vi "RecorderMain.vi"(2 "Timer (Timer 1)":T1 items=["Timer 1", "Timer 2", "Timer 3"], 5 "NXT":T2={"Hardware"="NXT", "Flattened String"=""}) -> ()   [LabVIEW 2010, in "Recorder.lvlib"]
uses:
  Recorder.lvlib
  <vilib>/NXT/Subs/LVHSConnector.ctl
  <vilib>/NXT/Block Support/NXT_TimerIndex.ctl
  <vilib>/NXT/Dual Mode Library/Waits/Wait_Num(msec).vi
  Components/Components.lvlib
panel:
  out "LastWriterPowers":i16[](array[numeric])
  out "TeleopEnabled":bool
  out "Stop Program?":bool
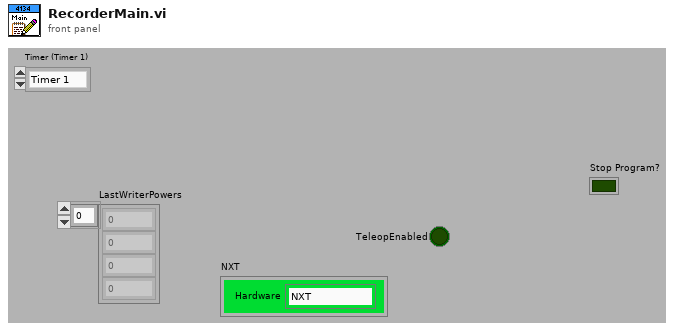
[diagram p1: front panel]
types:
  T1 = typedef "NXT_TimerIndex.ctl" = u8
  T2 = typedef "LVHSConnector.ctl" = cluster{"Hardware":string, "Flattened String":string}
  T3 = cluster{"FileName":string, "WriterEnabled?":bool, "TeleopEnabled?":bool, "StopProgram?":bool, "ArraySize":u8}
  T4 = typedef "NXT_FileStatusCodes.ctl" = u16
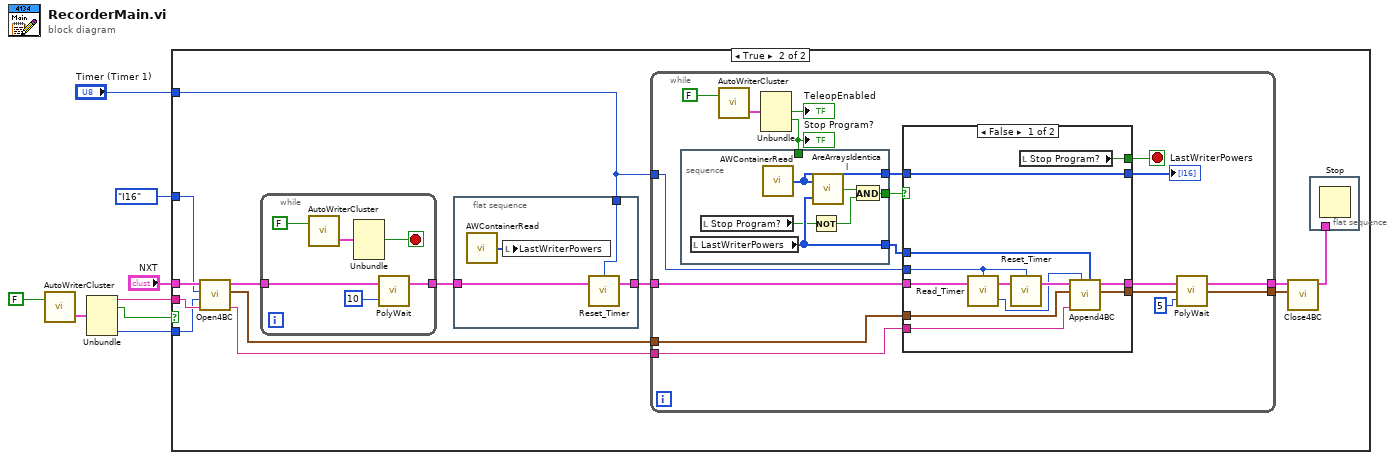
[diagram p0: block diagram]
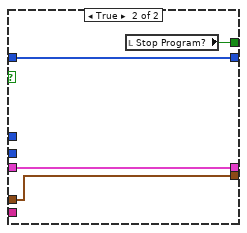
[diagram p3: hidden frame]
diagram:
  n1 = call "AutoWriterCluster.vi"("Mode(Write=True)"=FALSE) -> ("Output"=w7:T3)  [unwired: 1 in]
  n2 = Unbundle(w7) -> ("FileName"=w5:string, "WriterEnabled?"=w6:bool, "ArraySize"=w4:u8)  [unwired: 2 out]
  n3 = case shown="True" w6 {
    tunnel: w5 -> [_ w18]
    tunnel: w4 -> [_ w17]
    tunnel: "NXT" -> [_ w16]
    tunnel: "Timer (Timer 1)" -> [_ w15]
    tunnel: enum8{"I8", "I16"}."I16" ("Storage Size (I16)") -> [_ w10]
    frame False {
    }
    frame True {
      n4 = call "Open4BC.vi"("File"=w18, "Number Of Motors"=w17, "Storage Size (I16)"=w10, "NXT"=w16) -> ("Header"=w12:string, "File Information"=w13:cluster{"File Handle Out":u8, "Error out":T4}, "NXT"=w19:T2)  [unwired: 5 in]
      n5 = while {
        tunnel: w19 -> [w30]
        tunnel: [w29] -> w14
        stop <- w26 stop-if-true
        n6 = call "AutoWriterCluster.vi"("Mode(Write=True)"=FALSE) -> ("Output"=w27:T3)  [unwired: 1 in]
        n7 = Unbundle(w27) -> ("TeleopEnabled?"=w26:bool)  [unwired: 4 out]
        n8 = call-poly <vilib>:"PolyWait.vi"("Time (100 msec)"=u32 10 ("Time (msec)"), "NXT"=w30) -> ("NXT"=w29:T2)  [unwired: 2 in]
      }
      n9 = flat-sequence {
        tunnel: w14 -> [w23]
        tunnel: [w25] -> w21
        tunnel: w15 -> [w22]
        frame #0 {
          n10 = call "AWContainerRead.vi"() -> ("Output"=w24:i16[])  [unwired: 1 in]
          n11 = local write "LastWriterPowers"(w24) -> ()
          n12 = call <vilib>:"Reset_Timer.vi"("NXT"=w23, "Timer (Timer 1)"=w22) -> ("NXT"=w25:T2)  [unwired: 2 in]
        }
      }
      n13 = while {
        tunnel: [w34] -> w20
        tunnel: w13 -> [w48]
        tunnel: w12 -> [w47]
        tunnel: [w36] -> w11
        tunnel: w21 -> [w42]
        tunnel: w15 -> [w37]
        stop <- w43 stop-if-true
        n14 = call "AutoWriterCluster.vi"("Mode(Write=True)"=FALSE) -> ("Output"=w40:T3)  [unwired: 1 in]
        n15 = Unbundle(w40) -> ("TeleopEnabled?"=→"TeleopEnabled":bool, "StopProgram?"=w32:bool)  [unwired: 3 out]
        "Stop Program?" <- w32
        n16 = stacked-sequence {
          tunnel: [w53] -> w45
          tunnel: [w52] -> w44
          tunnel: [w51] -> w41
          tunnel: w32 -> [_]
          frame #0 {
            n17 = local read "LastWriterPowers"() -> (w52:i16[])
            n18 = local read "Stop Program?"() -> (w50:bool)
            n19 = call "AWContainerRead.vi"() -> ("Output"=w51:i16[])  [unwired: 1 in]
            n20 = Not(x=w50) -> (.not. x?=w49:bool)
            n21 = call "AreArraysIdentical.vi"("ArrayY"=w52, "ArrayX"=w51) -> ("Equal?"=w54:bool)  [unwired: 4 in]
            n22 = And(x=w54, y=w49) -> (x .and. y?=w53:bool)
          }
        }
        n23 = case shown="False" w45 {
          tunnel: w42 -> [w62 w70]
          tunnel: [w59 w70] -> w35
          tunnel: w48 -> [w55 w67]
          tunnel: w47 -> [w56 _]
          tunnel: [w66 w67] -> w36
          tunnel: [w65 w68] -> w46
          tunnel: w41 -> [w65 w68]
          tunnel: w44 -> [w64 _]
          tunnel: [w63 w69] -> w43
          tunnel: w37 -> [w57 _]
          frame False {
            n24 = call <vilib>:"Read_Timer.vi"("NXT"=w62, "Timer (Timer 1)"=w57) -> ("Value (msec)"=w58:u32, "NXT"=w61:T2)  [unwired: 1 in]
            n25 = call <vilib>:"Reset_Timer.vi"("NXT"=w61, "Timer (Timer 1)"=w57) -> ("NXT"=w60:T2)  [unwired: 2 in]
            n26 = local read "Stop Program?"() -> (w63:bool)
            n27 = call "Append4BC.vi"("Array"=w64, "Time"=w58, "Header"=w56, "File Information"=w55, "NXT"=w60) -> ("File Information"=w66:cluster{"File Handle Out":u8, "Error out":T4}, "NXT"=w59:T2)  [unwired: 5 in]
          }
          frame True {
            n28 = local read "Stop Program?"() -> (w69:bool)
          }
        }
        "LastWriterPowers" <- w46
        n29 = call-poly <vilib>:"PolyWait.vi"("Time (100 msec)"=u32 5, "NXT"=w35) -> ("NXT"=w34:T2)  [unwired: 2 in]
      }
      n30 = call "Close4BC.vi"("File Information"=w11, "NXT"=w20) -> ("NXT"=w9:T2)  [unwired: 9 in]
      n31 = flat-sequence {
        tunnel: w9 -> [_]
        frame #0 {
          n32 = Stop() -> ()  [unwired: 1 in]
        }
      }
    }
  }
